vi "LabVIEW Cluster Item Not Named Prefix.vi"() -> (0 "not named cluster item prefix":string="LVClusterItem_")   [LabVIEW 2014]
panel:
  # "Prefix stored in this VI as default value."
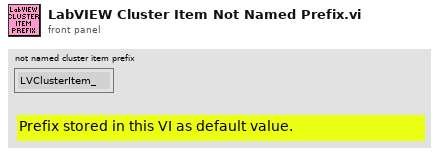
[diagram p1: front panel]
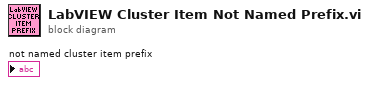
[diagram p0: block diagram]
diagram:
